vi "HTTP Server.vi"(11 "VolatusAPI in":refnum<class "VolatusAPI.lvclass">) -> (2 "HTTP":refnum<class "Server.lvclass">, 3 "VolatusAPI out":refnum<class "VolatusAPI.lvclass">)   [LabVIEW 2020, in "Volatus.lvlib" / "VolatusAPI.lvclass"]
uses:
  VolatusAPI.lvclass
  VolatusAPI.lvclass/VolatusAPI.ctl
  lv-vecto/Vecto/Vecto/Vecto.lvclass
  lv-http-server/HTTP Server/Server/Server.lvclass
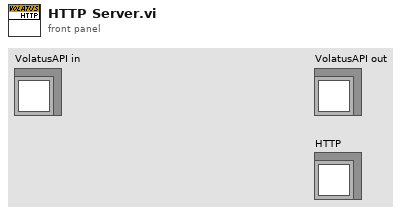
[diagram p1: front panel]
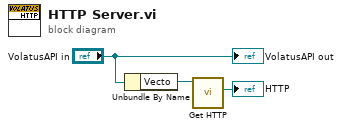
[diagram p0: block diagram]
diagram:
  n1 = Unbundle By Name("VolatusAPI in") -> ("Vecto"=w2:refnum<class "Vecto.lvclass">)
  n2 = call "Get HTTP.vi"("Vecto in"=w2) -> ("HTTP"=→"HTTP":refnum<class "Server.lvclass">)  [unwired: 8 in, 2 out]
  "VolatusAPI out" <- "VolatusAPI in"
